vi "GetGrowInfo.vi"(0 "XRef":T18, 1 "State In":T6={"Worker Library Path"=path "", "Block Label"="", "Types"=[], "Selections"=[], "Icon"={"image type"=0, "image depth"=0, "image"=[], "mask"=[], "colors"=[], "Rectangle"={"left"=0, "top"=0, "right"=0, "bottom"=0}}, "Errors"={"Terminals"=[], "Generate"={"status"=FALSE, "code"=0, "source"=""}}, "Calculated Sizes"={"Block Width"=0, "Block Height"=0, "Half Width"=0, "Icon Top"=0, "Icon Bottom"=0, "Label Width"=0, "Half Label"=0, "Label Top"=0, "Text Width"=0, "Half Text"=0, "Text Height"=0, "Label Height"=0, "Expanded Width"=0, "Label Bottom"=0, "Expanded Top"=0, "Expanded Bottom"=0, "Expanded Height"=0, "Min Height"=0, "Max Height"=0}, "Special Terminal Indices"={"Action"=-1, "Init"=-1, "Tag"=-1, "State in"=-1, "State out"=-1, "Error"=-1}, "Terminals"=[]}) -> (14 "Grow Info":T2, 15 "Fatal Error Out":T1)   [LabVIEW 2022 SP3, in "Flex Block.xnode"]
uses:
  Flex Block.xnode
  <vilib>/XNodeSupport/XNodeXNodeRef.ctl
  State.ctl
  FlexBlocks Support/Type Descriptor.ctl
  FlexBlocks Support/Terminal Direction.ctl
  FlexBlocks Support/Value Mode.ctl
  FlexBlocks Support/Special Terminal.ctl
  <vilib>/picture/picture.llb/imagedata.ctl
  FlexBlocks Support/XNode Errors.ctl
  FlexBlocks Support/Calculated Sizes.ctl
  FlexBlocks Support/Special Terminal Indices.ctl
  FlexBlocks Support/Terminal Status.ctl
  FlexBlocks Support/Terminal State.ctl
  FlexBlocks Support/Terminal Draw Style.ctl
  <vilib>/XNodeSupport/XNodeGrowInfo.ctl
  <vilib>/XNodeSupport/XNodeBounds.ctl
  <vilib>/XNodeSupport/XNodeInt.ctl
  <vilib>/XNodeSupport/XNodeBool.ctl
  <vilib>/XNodeSupport/XNodeErrorCluster.ctl
  <vilib>/XNodeSupport/NI_XNodeSupport.lvlib
  FlexBlocks Support/FlexBlocks Support.lvlib
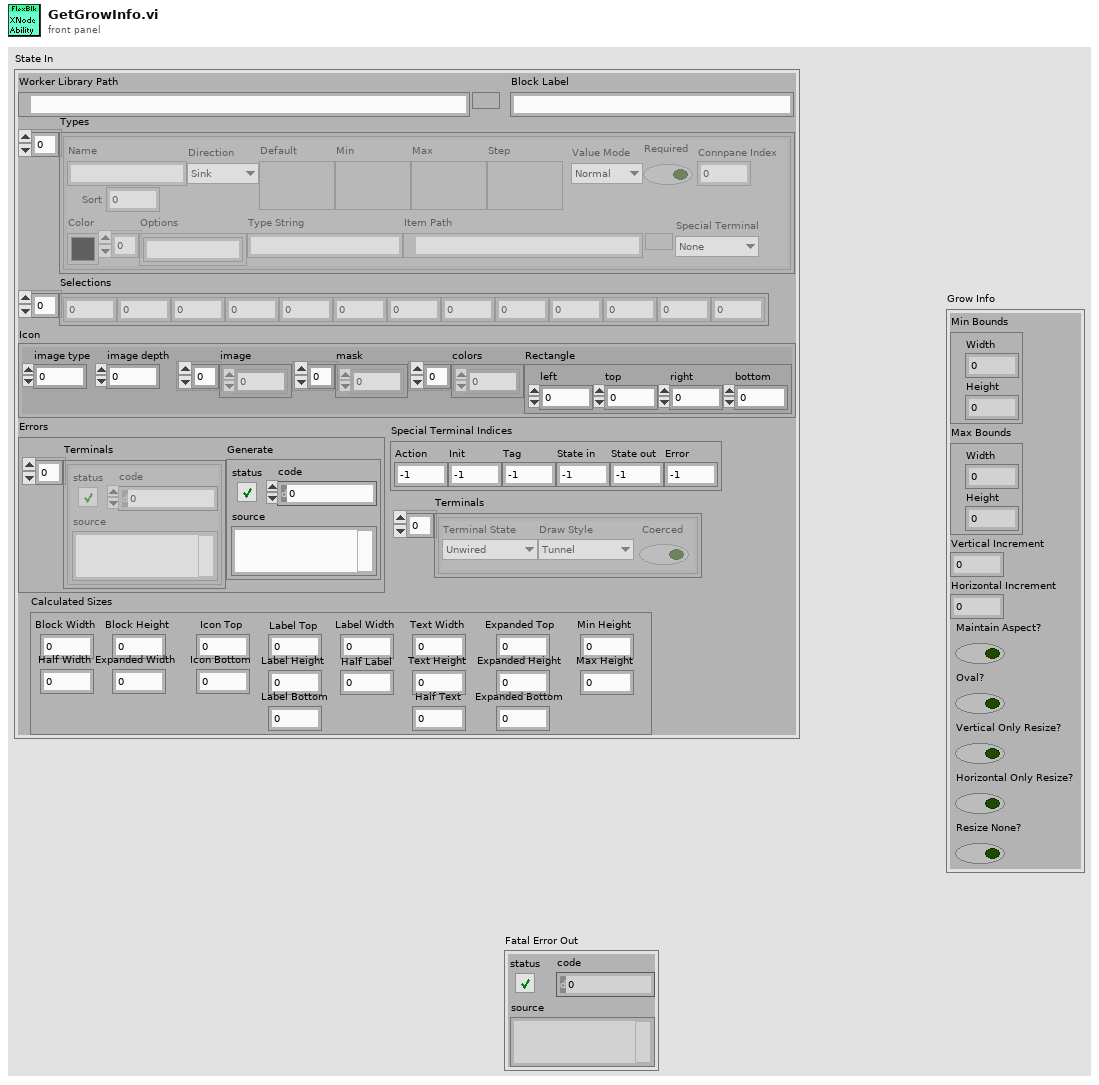
[diagram p1: front panel]
types:
  T1 = typedef "NI_XNodeSupport.lvlib/XNodeErrorCluster.ctl" = errorcluster
  T2 = typedef "NI_XNodeSupport.lvlib/XNodeGrowInfo.ctl" = cluster{"Min Bounds":T3, "Max Bounds":T3, "Vertical Increment":T4, "Horizontal Increment":T4, "Maintain Aspect?":T5, "Oval?":T5, "Vertical Only Resize?":T5, "Horizontal Only Resize?":T5, "Resize None?":T5}
  T3 = typedef "NI_XNodeSupport.lvlib/XNodeBounds.ctl" = cluster{"Width":T4, "Height":T4}
  T4 = typedef "NI_XNodeSupport.lvlib/XNodeInt.ctl" = i32
  T5 = typedef "NI_XNodeSupport.lvlib/XNodeBool.ctl" = bool
  T6 = typedef "Flex Block.xnode/State.ctl" = cluster{"Worker Library Path":path, "Block Label":string, "Types":T7[], "Selections":i32[], "Icon":T11, "Errors":T12, "Calculated Sizes":T13, "Special Terminal Indices":T14, "Terminals":T15[]}
  T7 = typedef "FlexBlocks Support.lvlib/Type Descriptor.ctl" = cluster{"Name":string, "Direction":T8, "Default":variant, "Min":variant, "Max":variant, "Step":variant, "Value Mode":T9, "Color":u32, "Options":string[], "Type String":string, "Item Path":path, "Required":bool, "Connpane Index":i32, "Special Terminal":T10, "Sort":i32}
  T8 = typedef "FlexBlocks Support.lvlib/Terminal Direction.ctl" = enum16{"Sink", "Source"}
  T9 = typedef "FlexBlocks Support.lvlib/Value Mode.ctl" = enum16{"Normal", "Range", "Select"}
  T10 = typedef "FlexBlocks Support.lvlib/Special Terminal.ctl" = enum16{"None", "Action", "Init", "Tag", "State in", "State out", "Error"}
  T11 = typedef "imagedata.ctl" = cluster{"image type":i32, "image depth":i32, "image":u8[], "mask":u8[], "colors":u32[], "Rectangle":cluster{"left":i16, "top":i16, "right":i16, "bottom":i16}}
  T12 = typedef "FlexBlocks Support.lvlib/XNode Errors.ctl" = cluster{"Terminals":errorcluster[], "Generate":errorcluster}
  T13 = typedef "FlexBlocks Support.lvlib/Calculated Sizes.ctl" = cluster{"Block Width":i32, "Block Height":i32, "Half Width":i32, "Icon Top":i32, "Icon Bottom":i32, "Label Width":i32, "Half Label":i32, "Label Top":i32, "Text Width":i32, "Half Text":i32, "Text Height":i32, "Label Height":i32, "Expanded Width":i32, "Label Bottom":i32, "Expanded Top":i32, "Expanded Bottom":i32, "Expanded Height":i32, "Min Height":i32, "Max Height":i32}
  T14 = typedef "FlexBlocks Support.lvlib/Special Terminal Indices.ctl" = cluster{"Action":i32, "Init":i32, "Tag":i32, "State in":i32, "State out":i32, "Error":i32}
  T15 = typedef "FlexBlocks Support.lvlib/Terminal Status.ctl" = cluster{"Terminal State":T16, "Draw Style":T17, "Coerced":bool}
  T16 = typedef "FlexBlocks Support.lvlib/Terminal State.ctl" = enum16{"Unwired", "BadType", "BadRef", "Channel", "Value", "Control Ref"}
  T17 = typedef "FlexBlocks Support.lvlib/Terminal Draw Style.ctl" = enum16{"Tunnel", "BadType", "BadRef", "Channel", "Value", "Control Ref"}
  T18 = typedef "NI_XNodeSupport.lvlib/XNodeXNodeRef.ctl" = refnum<vi>
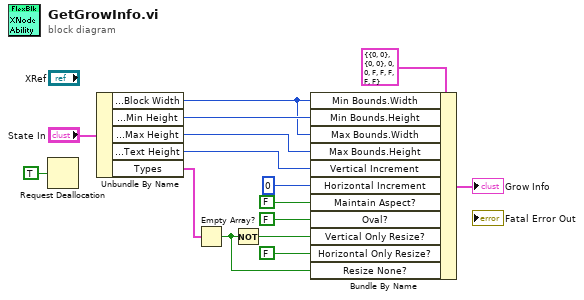
[diagram p0: block diagram]
diagram:
  n1 = Request Deallocation(TRUE ("flag")) -> ()
  n2 = Unbundle By Name("State In") -> ("Calculated Sizes.Block Width"=w11:i32, "Calculated Sizes.Min Height"=w12:i32, "Calculated Sizes.Max Height"=w10:i32, "Calculated Sizes.Text Height"=w5:i32, "Types"=w4:T7[])
  n3 = Empty Array?(array=w4) -> (empty?=w1:bool)
  n4 = Not(x=w1) -> (.not. x?=w2:bool)
  n5 = Bundle By Name(cluster=T2 {"Min Bounds"={"Width"=0, "Height"=0}, "Max Bounds"={"Width"=0, "Height"=0}, "Vertical Increment"=0, "Horizontal Increment"=0, "Maintain Aspect?"=FALSE, "Oval?"=FALSE, "Vertical Only Resize?"=FALSE, "Horizontal Only Resize?"=FALSE, "Resize None?"=FALSE} ("Grow Info"), "Min Bounds.Width"=w11, "Min Bounds.Height"=w12, "Max Bounds.Width"=w11, "Max Bounds.Height"=w10, "Vertical Increment"=w5, "Horizontal Increment"=T4 0, "Maintain Aspect?"=T5 FALSE, "Oval?"=T5 FALSE, "Vertical Only Resize?"=w2, "Horizontal Only Resize?"=T5 FALSE, "Resize None?"=w1) -> (→"Grow Info":T2)
